vi "check ack.vi"(8 "error in (no error)":errorcluster caption="에러 입력(에러 없음)", 10 "Read Data":u8[](array[numeric]), 11 "I2C 입력":refnum<class "I2C.lvclass">) -> (0 "error out":errorcluster caption="에러 출력", 2 "Read Data Out":u8[](array[numeric]), 3 "I2C 출력":refnum<class "I2C.lvclass">)   [LabVIEW 2020, in "I2C.lvclass"]
uses:
  I2C.lvclass
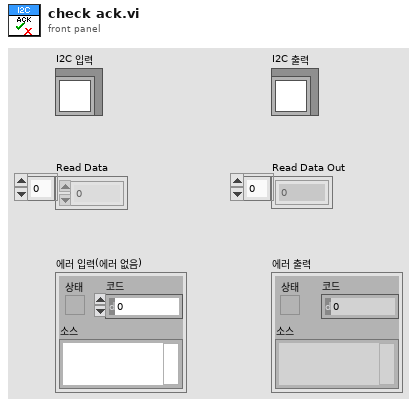
[diagram p1: front panel]
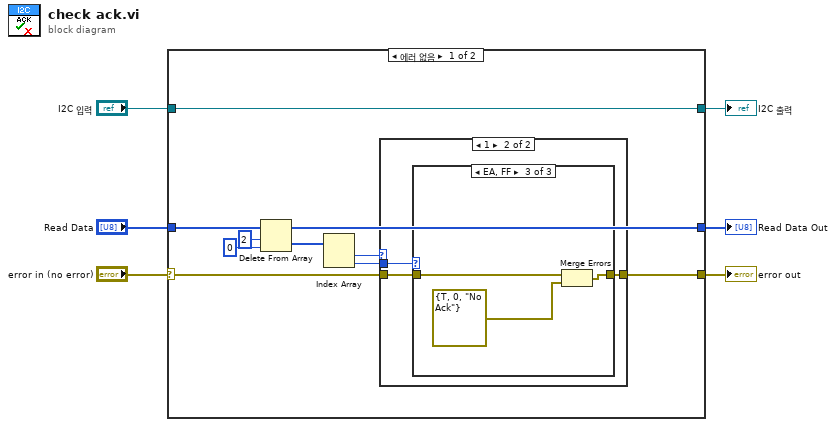
[diagram p0: block diagram]
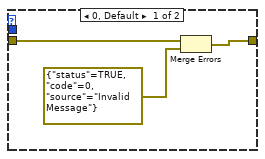
[diagram p2: hidden frame]
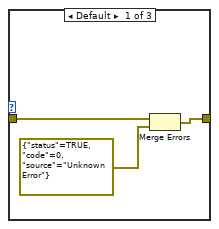
[diagram p3: hidden frame]
diagram:
  n1 = case shown="에러 없음" "error in (no error)" {
    selector: "error in (no error)" -> [w8 w32]
    tunnel: [w7 w32] -> w5
    tunnel: [w16 w31] -> w3
    tunnel: "I2C 입력" -> [w16 w31]
    tunnel: "Read Data" -> [w12 w30]
    tunnel: [w9 w30] -> w1
    frame No Error {
      n2 = Delete From Array(array=w12, length=2 ("길이"), index=0 ("인덱스")) -> (deleted portion=w15:u8[], array with subset deleted=w9:u8[])
      n3 = Index Array(array=w15) -> (element #1=w13:u8, element #2=w14:u8)  [unwired: 2 in]
      n4 = case shown="1" w13 {
        tunnel: [w18 w22] -> w7
        tunnel: w8 -> [w19 w21]
        tunnel: w14 -> [_ w20]
        frame 0, Default {
          n5 = Merge Errors(w19, errorcluster {"status"=TRUE, "code"=0, "source"="Invalid Message"} ("error IO")) -> (w18:errorcluster)
        }
        frame 1 {
          n6 = case shown="EA, FF" w20 {
            tunnel: w21 -> [w25 w26 w29]
            tunnel: [w24 w26 w28] -> w22
            frame Default {
              n7 = Merge Errors(w25, errorcluster {"status"=TRUE, "code"=0, "source"="Unknown Error"} ("에러 입력")) -> (w24:errorcluster)
            }
            frame 0..2, 16..18 {
              # "OK"
            }
            frame 234, 255 {
              n8 = Merge Errors(w29, errorcluster {"status"=TRUE, "code"=0, "source"="No Ack"} ("에러 입력")) -> (w28:errorcluster)
            }
          }
        }
      }
    }
    frame Error {
    }
  }
  "error out" <- w5
  "I2C 출력" <- w3
  "Read Data Out" <- w1
